vi "Load_Geometry_ColDet.vi"(8 "error in":errorcluster, 10 "Data Folder":path) -> (0 "error out":errorcluster, 1 "Number Moving":i32, 2 "Number Static":i32)   [LabVIEW 2011]
doc: "This VI is used to load in the relevant geometry for the tunnel model. The various models (and only those models!) should be read in from seperate folders. The probe folder should contain only the probe gemotery, a single .3DS file. The Static geometry is stationary and cannot be moved. The Moving geometry is movable through rotations and translations. .3DS files can be created in 3DS Max, a downloadable software that is free to students. Goto the autodesk website to download."
uses:
  Enflo_Collision_Detection.dll
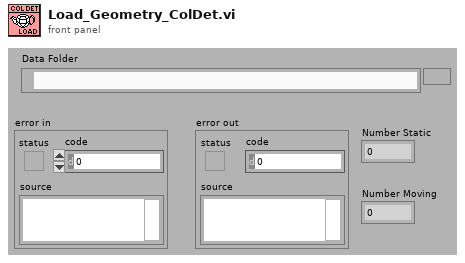
[diagram p1: front panel]
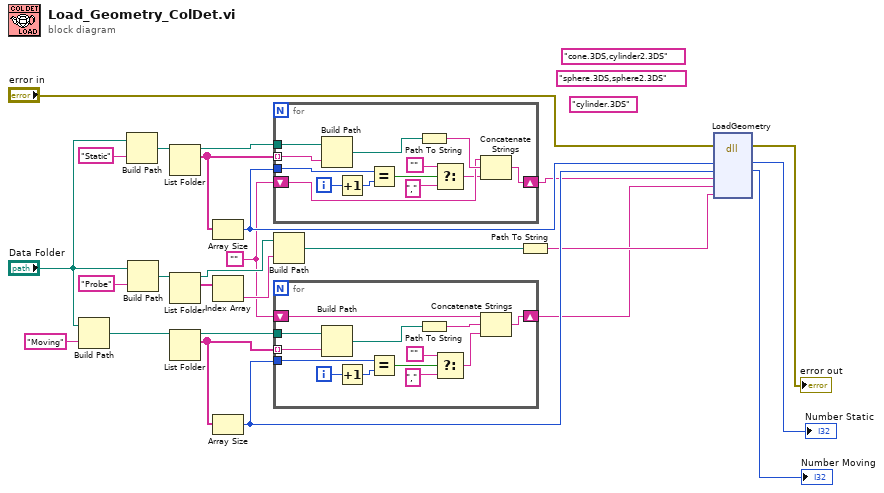
[diagram p0: block diagram]
diagram:
  (unwired) "sphere.3DS,sphere2.3DS" ("Moving Files")
  (unwired) "cone.3DS,cylinder2.3DS" ("Static Files")
  (unwired) "cylinder.3DS" ("Static Files")
  w13 = ""
  n1 = Build Path(base path="Data Folder", name or relative path="Moving") -> (appended path=w8:path)
  n2 = Build Path(base path="Data Folder", name or relative path="Static") -> (appended path=w4:path)
  n3 = Build Path(base path="Data Folder", name or relative path="Probe") -> (appended path=w6:path)
  n4 = List Folder(path=w4) -> (path out=w18:path, filenames=w19:string[])  [unwired: 3 in, 2 out]
  n5 = List Folder(path=w6) -> (path out=w20:path, filenames=w23:string[])  [unwired: 3 in, 2 out]
  n6 = List Folder(path=w8) -> (path out=w15:path, filenames=w14:string[])  [unwired: 3 in, 2 out]
  n7 = Array Size(array=w19) -> (size(s)=w17:i32)
  n8 = Index Array(array=w23) -> (element=w22:string)  [unwired: 1 in]
  n9 = Array Size(array=w14) -> (size(s)=w16:i32)
  n10 = for {
    tunnel: w19 -> [w37] mode=indexing
    tunnel: w18 -> [w38]
    shift-right: [w33] -> w3
    shift-left: w13 -> [w34]
    tunnel: w17 -> [w32]
    i -> [w31]
    n11 = Build Path(base path=w38, name or relative path=w37) -> (appended path=w36:path)
    n12 = Increment(x=w31) -> (x+1=w26:i32)
    n13 = Equal?(x=w32, y=w26) -> (x = y?=w30:bool)
    n14 = Path To String(path=w36) -> (string=w35:string)
    n15 = Select(t="", s=w30, f="," ("string")) -> (s? t:f=w28:string)
    n16 = Concatenate Strings(w34, w35, w28) -> (w33:string)
  }
  n17 = Build Path(base path=w20, name or relative path=w22) -> (appended path=w21:path)
  n18 = for {
    tunnel: w14 -> [w50] mode=indexing
    tunnel: w15 -> [w51]
    shift-right: [w46] -> w1
    shift-left: w13 -> [w47]
    tunnel: w16 -> [w45]
    i -> [w44]
    n19 = Build Path(base path=w51, name or relative path=w50) -> (appended path=w49:path)
    n20 = Increment(x=w44) -> (x+1=w39:i32)
    n21 = Equal?(x=w45, y=w39) -> (x = y?=w43:bool)
    n22 = Path To String(path=w49) -> (string=w48:string)
    n23 = Select(t="", s=w43, f="," ("string")) -> (s? t:f=w41:string)
    n24 = Concatenate Strings(w47, w48, w41) -> (w46:string)
  }
  n25 = Path To String(path=w21) -> (string=w2:string)
  n26 = dll-call lib="C:/Users/Nick Martin/Desktop/Release/Release/Enflo_Collision_Detection.dll" fn="LoadGeometry"(error in="error in", "Number Static"=w17, "Number Moving"=w16, "Static Files"=w3, "Moving Files"=w1, "Probe File"=w2) -> (error out=→"error out":errorcluster, "Number Static"=→"Number Static":i32, "Number Moving"=→"Number Moving":i32)  [unwired: 6 in, 1 out]
